vi "Cast Device Status.vi"(11 "register values":u16[](array[numeric])) -> (2 "Invalid Data":bool[](array[boolean]), 3 "Connected":bool[](array[boolean]))   [LabVIEW 2024, in "IOLink.lvlib"]
uses:
  IOLink.lvlib
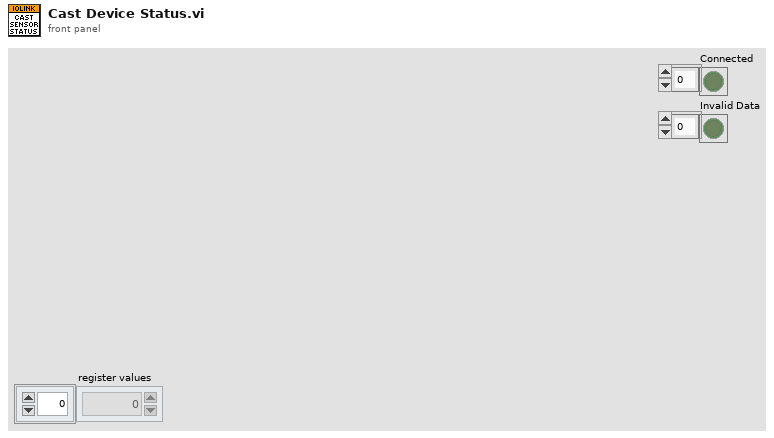
[diagram p1: front panel]
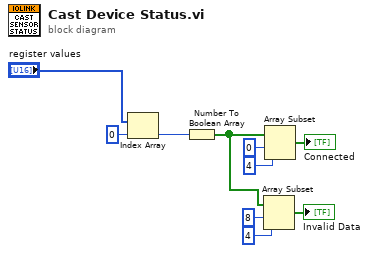
[diagram p0: block diagram]
diagram:
  n1 = Index Array(array="register values", index=0) -> (element=w9:u16)
  n2 = Number To Boolean Array(number=w9) -> (Boolean array=w4:bool[])
  n3 = Array Subset(array=w4, index=8, length=4) -> (→"Invalid Data":bool[])
  n4 = Array Subset(array=w4, index=0, length=4) -> (→"Connected":bool[])
